vi "test Random (0 - 1) with Seed.vi"(8 "error in (no error)":errorcluster, 11 "TestCase in":refnum<class "Position Estimation Tests.lvclass">) -> (0 "error out":errorcluster, 3 "TestCase out":refnum<class "Position Estimation Tests.lvclass">)   [LabVIEW 2014, in "Utility VIs tests.lvclass"]
uses:
  Utility VIs tests.lvclass
  Position Estimation Tests/Position Estimation Tests.lvclass
  SPLAT/Global_seed.vi
  <vilib>/addons/_JKI Toolkits/VI Tester/TestCase.llb/TestCase.lvclass
  SPLAT/Tag.lvclass
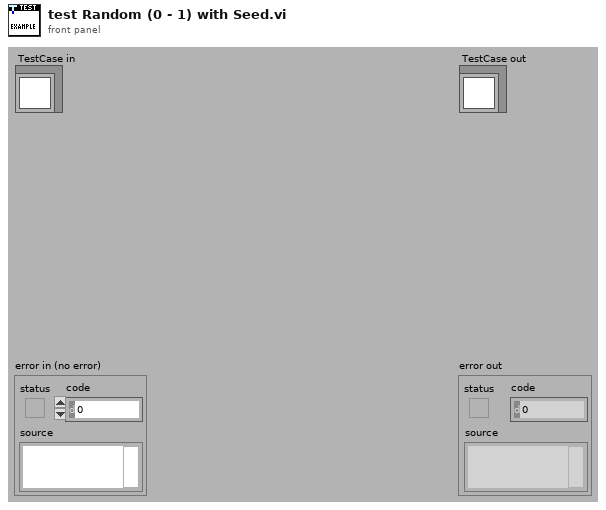
[diagram p1: front panel]
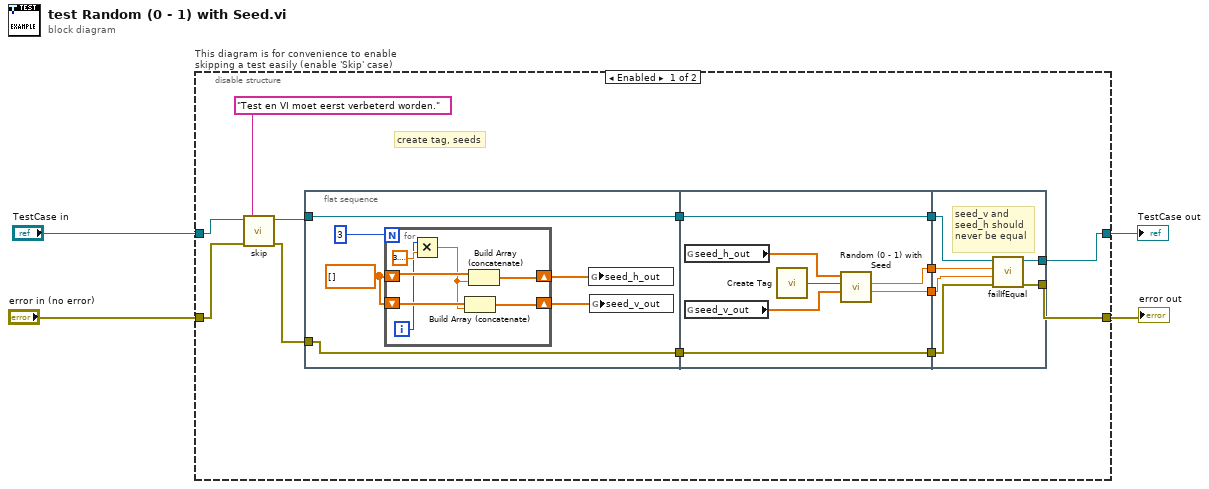
[diagram p0: block diagram]
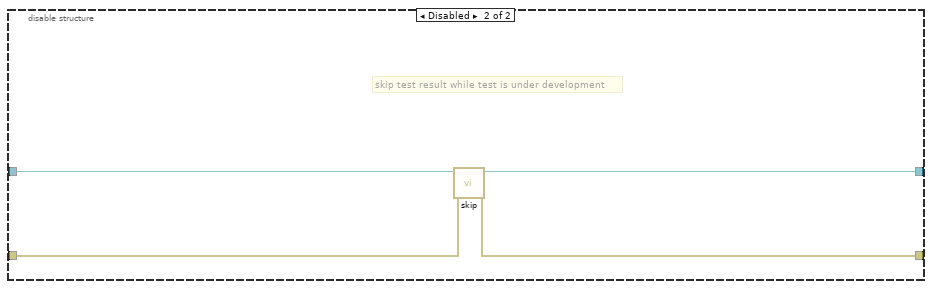
[diagram p2: hidden frame]
diagram:
  n1 = disable-structure "This diagram is for convenience to enable skipping a test easily (enable 'Skip' case)" shown="Enabled" {
    disable-tunnel: "TestCase in" -> [w9 w47]
    disable-tunnel: [w12 w45] -> w2
    disable-tunnel: [w13 w46] -> w3
    disable-tunnel: "error in (no error)" -> [w7 w44]
    frame Enabled {
      # "create tag, seeds"
      n2 = call <vilib>:"skip.vi"("error in (no error)"=w7, "skipMessage"="Test en VI moet eerst verbeterd worden.", "TestCase in"=w9) -> ("error out"=w6:errorcluster, "TestCase out"=w8:refnum<class "Position Estimation Tests.lvclass">)  [unwired: 7 in]
      n3 = flat-sequence {
        tunnel: w8 -> [w19]
        tunnel: [w19] -> w16
        tunnel: w6 -> [w18]
        tunnel: [w18] -> w14
        tunnel: [w34] -> w17
        tunnel: w16 -> [w34]
        tunnel: [w33] -> w15
        tunnel: w14 -> [w33]
        tunnel: [w32] -> w11
        tunnel: [w31] -> w10
        tunnel: w17 -> [w43]
        tunnel: w15 -> [w42]
        tunnel: [w41] -> w13
        tunnel: [w40] -> w12
        tunnel: w11 -> [w39]
        tunnel: w10 -> [w38]
        frame #0 {
          w21 = dbl[] []
          n4 = for {
            N: 3 -> [_]
            shift-right: [w29] -> w22
            shift-left: w21 -> [w28]
            shift-right: [w26] -> w20
            shift-left: w21 -> [w27]
            i -> [w24]
            n5 = Multiply(x=w24, y=3.141592653589793) -> (x*y=w25:dbl)
            n6 = Build Array (concatenate)(w27, w25) -> (w26:dbl[])
            n7 = Build Array (concatenate)(w28, w25) -> (w29:dbl[])
          }
          n8 = global write "Global_seed.vi" "seed_h_out"(w22) -> ()
          n9 = global write "Global_seed.vi" "seed_v_out"(w20) -> ()
        }
        frame #1 {
          n10 = global read "Global_seed.vi" "seed_h_out"() -> (w36:dbl[])
          n11 = global read "Global_seed.vi" "seed_v_out"() -> (w35:dbl[])
          n12 = call "Create Tag.vi"() -> ("Tag Out"=w37:refnum<class "Tag.lvclass">)  [unwired: 3 in]
          n13 = call "Random (0 - 1) with Seed.vi"("v_seeds_in"=w35, "Tag.lvclass"=w37, "h_seeds_in"=w36) -> ("v_element"=w31:dbl, "h_element"=w32:dbl)  [unwired: 5 in, 2 out]
        }
        frame #2 {
          # "seed_v and\nseed_h should \nnever be equal"
          n14 = call-dynamic "failIfEqual.vi"("error in (no error)"=w42, "y"=w38, "x"=w39, "TestCase in"=w43) -> ("error out"=w41:errorcluster, "TestCase out"=w40:refnum<class "Position Estimation Tests.lvclass">)  [unwired: 6 in]
        }
      }
    }
    frame Disabled {
      # "skip test result while test is under development"
      n15 = call <vilib>:"skip.vi"("error in (no error)"=w44, "TestCase in"=w47) -> ("error out"=w46:errorcluster, "TestCase out"=w45:refnum<class "Position Estimation Tests.lvclass">)  [unwired: 8 in]
    }
  }
  "error out" <- w3
  "TestCase out" <- w2
